vi "Write Image Msg.vi"(8 "error in (no error)":errorcluster, 10 "Image Acquisition.lvlib:Image Msg.lvclass":refnum<class "Image Msg.lvclass">, 11 "Image Acquisition in":refnum<class "Image Acquisition.lvclass">) -> (0 "error out":errorcluster, 3 "Image Acquisition out":refnum<class "Image Acquisition.lvclass">)   [LabVIEW 2016, in "Image Acquisition.lvlib" / "Image Acquisition.lvclass"]
uses:
  Image Acquisition.lvclass
  Image Acquisition Messages/Image Msg/Image Msg.lvclass
  Image Acquisition.lvclass/Image Acquisition.ctl
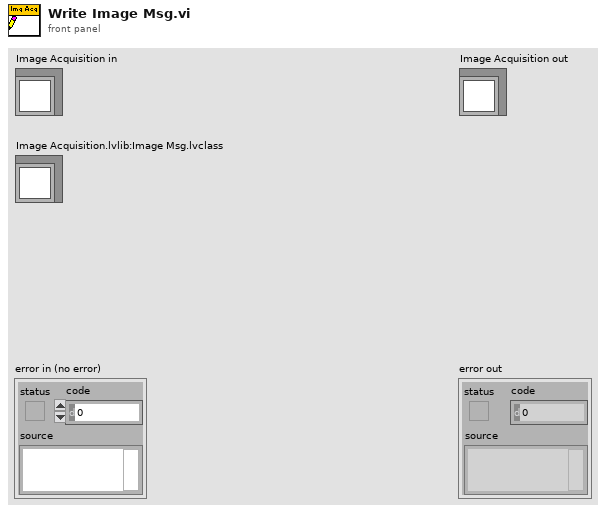
[diagram p1: front panel]
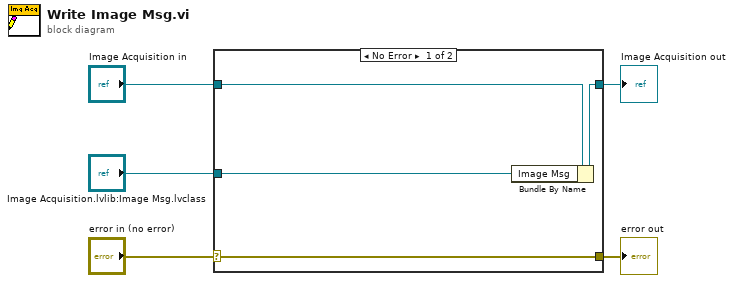
[diagram p0: block diagram]
diagram:
  n1 = case shown="No Error" "error in (no error)" {
    selector: "error in (no error)" -> [w9 w10]
    tunnel: [w9 w10] -> w4
    tunnel: [w7 w11] -> w2
    tunnel: "Image Acquisition in" -> [w8 w11]
    tunnel: "Image Acquisition.lvlib:Image Msg.lvclass" -> [w6 _]
    frame No Error {
      n2 = Bundle By Name(cluster=w8, "Image Msg"=w6) -> (w7:refnum<class "Image Acquisition.lvclass">)
    }
    frame Error {
    }
  }
  "error out" <- w4
  "Image Acquisition out" <- w2
